vi "set datatype.vi"(8 "error in (no error)":errorcluster, 10 "datatype":T1, 11 "JSON Helper in":refnum<class "JSON Value.lvclass">) -> (0 "error out":errorcluster, 3 "JSON Helper out":refnum<class "JSON Value.lvclass">)   [LabVIEW 2016, in "JSON Value.lvclass"]
uses:
  JSON Value.lvclass
  JSON Types.ctl
  JSON Value.lvclass/JSON Value.ctl
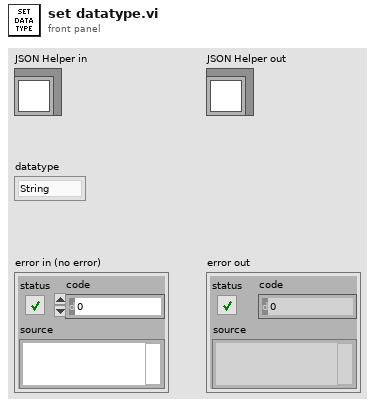
[diagram p1: front panel]
types:
  T1 = typedef "JSON Value.lvclass/JSON Types.ctl" = enum8{"String", "Numeric", "Boolean", "NULL", "Object", "Array"}
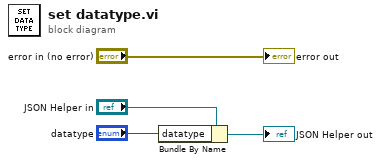
[diagram p0: block diagram]
diagram:
  n1 = Bundle By Name(cluster="JSON Helper in", "datatype"="datatype") -> (→"JSON Helper out":refnum<class "JSON Value.lvclass">)
  "error out" <- "error in (no error)"
